vi "LCVR Voltages Global 2015-Apr-07.vi"() -> ()   [LabVIEW 2014]
panel:
  in  "Current Wavelength (nm)":dbl=1083.0 format="%_7g"
  in  "SCD Wavelength Offsets (nm)":dbl[][](array[numeric])=[[0.2232, 0.2498, 0.2535, 0.2922, 0.3154, 0.5572, 0.5565, 0.0465, -0.766], [0.0272, -0.0023, -0.0032, -0.0034, -0.0038, -0.0073, -0.0044, -0.0061, 0.0194], [0.0021, 0.0194, 0.022, 0.0219, 0.0207, 0.0291, 0.0277, 0.0232, 0.0499], [0.0062, 0.0072, 0.0077, 0.0115, 0.0103, 0.0175, 0.0096, 0.0058, 0.031], [0.0, 0.0, 0.0, 0.0, 0.0, 0.0, 0.0, 0.0, 0.0]] min=-1.0 max=1.0 step=0.001 format="%.4f"
  out "SCD Fit Coefficients":dbl[][][](array[numeric])=[[[782150.642, 1241.61667, 0.77009403, 0.82470794, -0.88686004, 1.09197591, -1.23483817], [768303.733, 1215.85833, 0.76198568, 0.83135456, -0.89393177, 1.09226555, -1.27323258], [767687.55, 1214.225, 0.75122913, 0.82275499, -0.90681899, 1.09315255, -1.3061442], [752913.042, 1188.34167, 0.81803722, 0.83336103, -0.83627164, 1.08919016, -1.0297424], [745126.267, 1170.61667, 0.73953504, 0.82580951, -0.92066751, 1.09388617, -1.36403359], [710913.333, 1111.89167, 0.80743954, 0.82925548, -0.85066692, 1.09030038, -1.06205853], [710052.192, 1110.725, 0.81470202, 0.84440394, -0.8406569, 1.08936045, -1.06214031], [709008.55, 1108.725, 0.80389698, 0.81943407, -0.85485271, 1.09053576, -1.06261175], [697355.2, 1079.95, 0.797354, 0.83460732, -0.86087288, 1.09100256, -1.09119125]], [[1563852.843, 1134.27143, 0.7292645, 0.63649838, -0.9251264, 1.0940782, -1.20033886], [1536313.829, 1110.77143, 0.75369147, 0.6487408, -0.89876187, 1.09249769, -1.11714563], [1534470.271, 1109.84286, 0.74184453, 0.63751492, -0.9125396, 1.09347142, -1.14370388], [1505080.243, 1085.28571, 0.73110064, 0.64669132, -0.92267167, 1.09380854, -1.20502678], [1489231.986, 1074.55714, 0.771239, 0.6327106, -0.88326132, 1.09219185, -0.99488819], [1421456.071, 1020.28571, 0.76847275, 0.64357798, -0.8854632, 1.09229497, -1.01416362], [1420575.771, 1017.34286, 0.76974841, 0.67849424, -0.88010041, 1.0912961, -1.08572714], [1418415.071, 1014.12857, 0.78398378, 0.68098145, -0.86462796, 1.09035738, -1.03100873], [1393926.386, 989.11429, 0.72150416, 0.64409046, -0.93487192, 1.09471876, -1.22664317]], [[3133890.65, 1394.75, 0.71527505, 1.24150193, -1.02871099, 1.10488737, -1.7634769], [3072132.45, 1363.68333, 0.70966824, 1.24332149, -1.03545327, 1.10522842, -1.79021756], [3069621.05, 1362.96667, 0.70783051, 1.23123389, -1.03861882, 1.10568895, -1.76949584], [3009960.983, 1332.18333, 0.71207439, 1.23597817, -1.03415053, 1.10548799, -1.75448217], [2978738.883, 1316.18333, 0.71739215, 1.23797226, -1.02943262, 1.10537049, -1.72964535], [2842129.567, 1244.36667, 0.71974165, 1.24493378, -1.02833196, 1.10545007, -1.71973917], [2840322.433, 1242.68333, 0.69617456, 1.23726047, -1.05353682, 1.10672205, -1.8059356], [2835935.183, 1237.53333, 0.70834011, 1.23818036, -1.04135649, 1.10611081, -1.76018148], [2787958.817, 1204.46667, 0.73441606, 1.26361563, -1.01072981, 1.10411495, -1.70698846]], [[6277945.62, 1275.42, 0.81276074, 0.90214899, -0.84050561, 1.08889071, -1.16539963], [6144887.8, 1248.7, 0.81874159, 0.88914098, -0.83645892, 1.08896497, -1.10241923], [6145130.26, 1247.14, 0.80731338, 0.88458105, -0.84875328, 1.08976058, -1.14349594], [6021225.52, 1221.02, 0.79875685, 0.88154419, -0.85836526, 1.09044072, -1.16945536], [5965053.76, 1206.46, 0.80239987, 0.88787501, -0.85340226, 1.08999093, -1.16992646], [5693265.94, 1139.48, 0.78534823, 0.87929368, -0.87484074, 1.09150446, -1.22307251], [5687080.94, 1138.26, 0.79549344, 0.88340601, -0.8635539, 1.09079849, -1.18340063], [5670483.6, 1134.46, 0.82016286, 0.89364024, -0.83561435, 1.08892513, -1.10503266], [5583046.38, 1104.42, 0.83882176, 0.91261091, -0.81588496, 1.08783163, -1.06784607]], [[12632312.14, 1230.3, 0.76059061, 0.75494066, -0.89755109, 1.09288031, -1.1843643], [12289772.9, 1201.32, 0.8194035, 0.80685768, -0.83022655, 1.08805653, -1.05231073], [12280844.2, 1200.24, 0.79122436, 0.80111782, -0.85987038, 1.08984748, -1.15247493], [12038733.68, 1174.02, 0.75743588, 0.78222774, -0.89785424, 1.09239802, -1.25474606], [11916807.62, 1163.18, 0.78669943, 0.79522284, -0.86608301, 1.0905359, -1.14336109], [11373077.46, 1102.22, 0.80668596, 0.81720623, -0.8449571, 1.08920631, -1.0858078], [11365032.6, 1100.86, 0.84792633, 0.82413223, -0.80066543, 1.08657492, -0.92351242], [11344035.58, 1086.2, 0.77750583, 0.78510867, -0.87944727, 1.09149165, -1.18775497], [11155856.3, 1058.5, 0.87245966, 0.80521791, -0.77568256, 1.08537456, -0.86560187]]] format="%_9f"
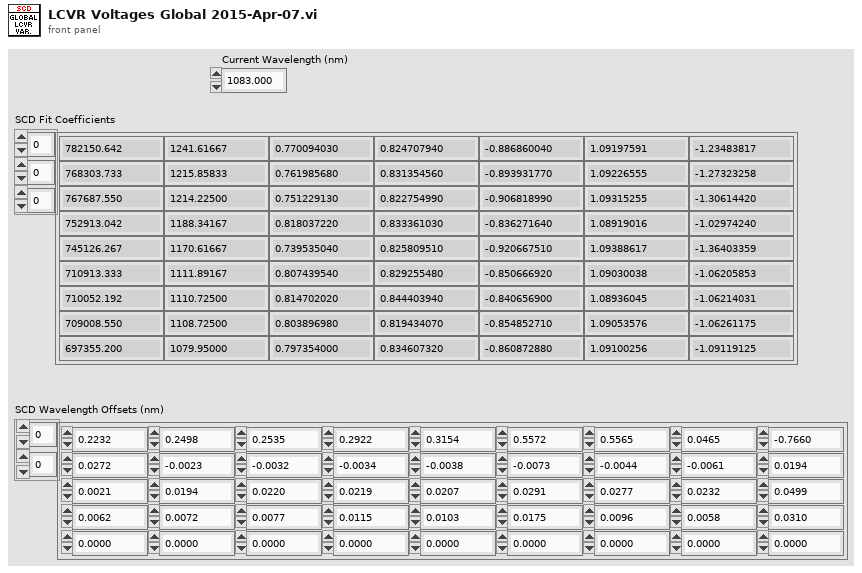
[diagram p1: front panel]
diagram:
